vi "get_signals_by_name.vi"(1 "Signals to read":refnum<k21>[](array[refnum]), 2 "Signal list":refnum<k21>[](array[refnum]), 3 "Signal data":dbl[](array[numeric])) -> (0 "Signals":dbl[](array[numeric]))   [LabVIEW 2017]
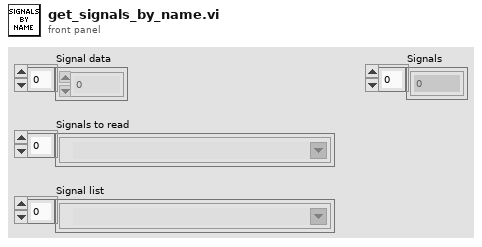
[diagram p1: front panel]
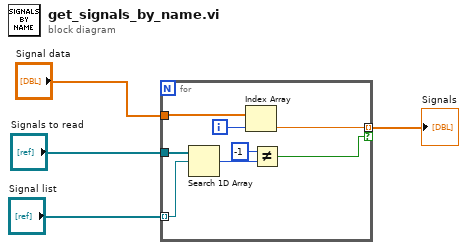
[diagram p0: block diagram]
diagram:
  n1 = for {
    tunnel: "Signals to read" -> [w5]
    tunnel: "Signal data" -> [w9]
    tunnel: "Signal list" -> [w6] mode=indexing
    tunnel: [w8] -> w4 mode=indexing if=w7
    i -> [w10]
    n2 = Search 1D Array(1D array=w5, element=w6) -> (index of element=w12:i32)  [unwired: 1 in]
    n3 = Index Array(array=w9, index=w10) -> (element=w8:dbl)
    n4 = Not Equal?(x=-1, y=w12) -> (x != y?=w7:bool)
  }
  "Signals" <- w4
